vi "V_on.vi"(1 "board_sel":u32=1) -> ()   [LabVIEW 2015]
uses:
  ESLSCDLL.dll
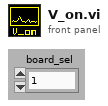
[diagram p1: front panel]
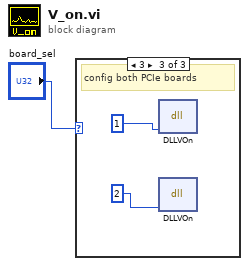
[diagram p0: block diagram]
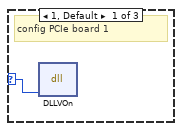
[diagram p2: hidden frame]
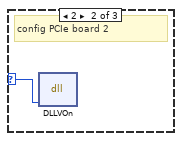
[diagram p3: hidden frame]
diagram:
  n1 = case shown="3" "board_sel" {
    selector: "board_sel" -> [w2 w3 _]
    frame 1, Default {
      # "config PCIe board 1"
      n2 = dll-call lib="C:/ENTW/PCIE/64bit/lv64/board.vis/ESLSCDLL.dll" fn="DLLVOn"("drv"=w2) -> ()  [unwired: 5 in, 2 out]
    }
    frame 2 {
      # "config PCIe board 2"
      n3 = dll-call lib="C:/ENTW/PCIE/64bit/lv64/board.vis/ESLSCDLL.dll" fn="DLLVOn"("drv"=w3) -> ()  [unwired: 5 in, 2 out]
    }
    frame 3 {
      # "config both PCIe boards"
      n4 = dll-call lib="C:/ENTW/PCIE/64bit/lv64/board.vis/ESLSCDLL.dll" fn="DLLVOn"("drv"=u32 1) -> ()  [unwired: 5 in, 2 out]
      n5 = dll-call lib="C:/ENTW/PCIE/64bit/lv64/board.vis/ESLSCDLL.dll" fn="DLLVOn"("drv"=u32 2) -> ()  [unwired: 5 in, 2 out]
    }
  }
